vi "call dll example.vi"() -> ()   [LabVIEW 2015]
uses:
  build/PwrXtalCal.dll
panel:
  out "error out":errorcluster
  out "result":dbl=-18.43
  in  "Freq":dbl=2412000000.0
  in  "RL":dbl
  in  "PhyPort":u16=6
  in  "PwrFreq":u16
  in  "VISA Resource Name":string="TCPIP0::10.144.41.39::inst0::INSTR"
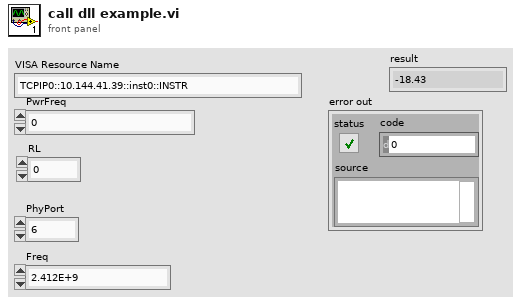
[diagram p1: front panel]
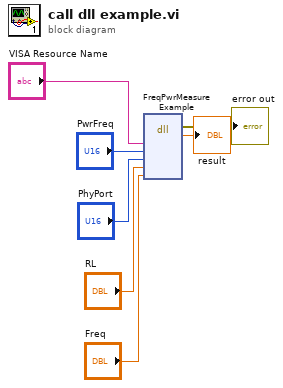
[diagram p0: block diagram]
diagram:
  n1 = dll-call lib="D:/WTM and WTS training/PwrXtalCalDLL/build/PwrXtalCal.dll" fn="FreqPwrMeasureExample"("VISA Resource Name"="VISA Resource Name", "PwrFreq"="PwrFreq", "PhyPort"="PhyPort", "RL"="RL", "Freq"="Freq") -> (error out=→"error out":errorcluster, "result"=→"result":dbl)  [unwired: 8 in, 1 out]
